vi "GetScanMoveType.vi"(11 "Scan Mode":T4) -> (1 "Detector":T1, 2 "Move Type":T2=enum."Continuous", 3 "Scan Type":T3=enum."Point")   [LabVIEW 2012]
uses:
  typedefs/ScanMode.ctl
  typedefs/Scan Type.ctl
  typedefs/Move Type.ctl
  typedefs/DetectorType.ctl
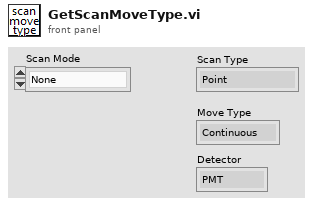
[diagram p1: front panel]
types:
  T1 = typedef "DetectorType.ctl" = enum16{"PMT", "SpectraWiz"}
  T2 = typedef "Move Type.ctl" = enum16{"None", "Continuous", "Discrete"}
  T3 = typedef "Scan Type.ctl" = enum16{"None", "Point", "Full Image Continuous", "Full Image Grab"}
  T4 = typedef "ScanMode.ctl" = enum16{"None", "Continuous", "Point Scan (CH3 cursor)", "Point Scan Move (CH3 cursor)", "Grab", "Grab Move Stage", "Grab Move Z-stage", "Cont. Move Z-stage", "Spec Move Stage", "Spec Move Cont", "Surf Calib"}
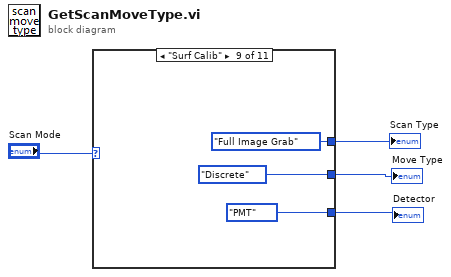
[diagram p0: block diagram]
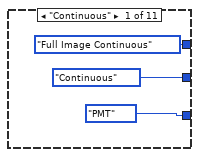
[diagram p2: hidden frame]
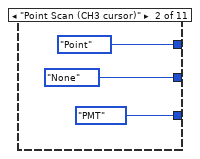
[diagram p3: hidden frame]
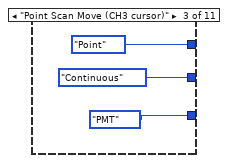
[diagram p4: hidden frame]
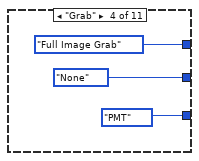
[diagram p5: hidden frame]
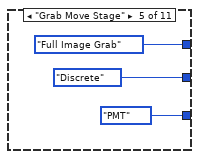
[diagram p6: hidden frame]
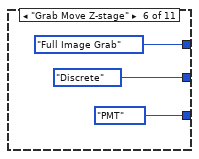
[diagram p7: hidden frame]
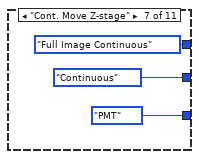
[diagram p8: hidden frame]
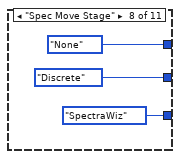
[diagram p9: hidden frame]
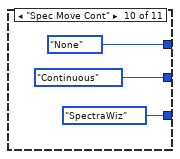
[diagram p10: hidden frame]
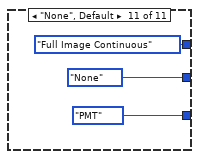
[diagram p11: hidden frame]
diagram:
  n1 = case shown="\"Surf Calib\"" "Scan Mode" {
    tunnel: [Scan_Type."Full Image Continuous" ("Scan Type") Scan_Type."Point" ("Scan Type") Scan_Type."Point" ("Scan Type") Scan_Type."Full Image Grab" ("Scan Type") Scan_Type."Full Image Grab" ("Scan Type") Scan_Type."Full Image Grab" ("Scan Type") Scan_Type."Full Image Continuous" ("Scan Type") Scan_Type."None" ("Scan Type") Scan_Type."Full Image Grab" ("Scan Type") Scan_Type."None" ("Scan Type") Scan_Type."Full Image Continuous" ("Scan Type")] -> w3
    tunnel: [Move_Type."Continuous" ("Move Type") Move_Type."None" ("Move Type") Move_Type."Continuous" ("Move Type") Move_Type."None" ("Move Type") Move_Type."Discrete" ("Move Type") Move_Type."Discrete" ("Move Type") Move_Type."Continuous" ("Move Type") Move_Type."Discrete" ("Move Type") Move_Type."Discrete" ("Move Type") Move_Type."Continuous" ("Move Type") Move_Type."None" ("Move Type")] -> w2
    tunnel: [DetectorType."PMT" ("Detector") DetectorType."PMT" ("Detector") DetectorType."PMT" ("Detector") DetectorType."PMT" ("Detector") DetectorType."PMT" ("Detector") DetectorType."PMT" ("Detector") DetectorType."PMT" ("Detector") DetectorType."SpectraWiz" ("Detector") DetectorType."PMT" ("Detector") DetectorType."SpectraWiz" ("Detector") DetectorType."PMT" ("Detector")] -> w1
    frame "Continuous" {
    }
    frame "Point Scan (CH3 cursor)" {
    }
    frame "Point Scan Move (CH3 cursor)" {
    }
    frame "Grab" {
    }
    frame "Grab Move Stage" {
    }
    frame "Grab Move Z-stage" {
    }
    frame "Cont. Move Z-stage" {
    }
    frame "Spec Move Stage" {
    }
    frame "Surf Calib" {
    }
    frame "Spec Move Cont" {
    }
    frame "None", Default {
    }
  }
  "Scan Type" <- w3
  "Move Type" <- w2
  "Detector" <- w1
